vi "Untitled 7 (SubVI).vi"(8 "dilution":dbl, 9 "fuel":dbl, 10 "primery air":dbl, 11 "w_t_dot":dbl) -> (2 "wt":dbl)   [LabVIEW 2019]
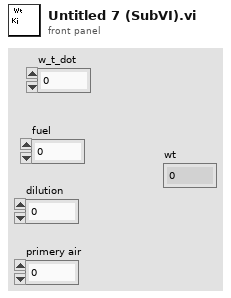
[diagram p1: front panel]
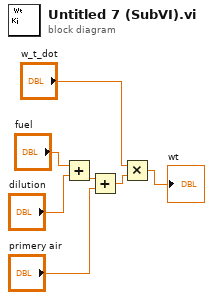
[diagram p0: block diagram]
diagram:
  n1 = Add(x="fuel", y="dilution") -> (x+y=w5:dbl)
  n2 = Add(x=w5, y="primery air") -> (x+y=w3:dbl)
  n3 = Multiply(x="w_t_dot", y=w3) -> (x*y=→"wt":dbl)
